vi "Single_ended_2575_DMM_handshake_scan.vi"(0 "resource name":refnum<k15>="R_signal", 1 "resource name":refnum<k15>="DMM", 2 "data path":path, 4 "Scan array":bool[][](array[boolean]), 5 "error in (no error)":errorcluster {"code" format="%.0x"}, 6 "Differential\nMode":bool, 7 "measurement type":T2, 11 "Resolution in Digits":T1=7.5 items=["3 1/2"=3.5, "4 1/2"=4.5, "5 1/2"=5.5, "6 1/2"=6.5, "7 1/2"=7.5], 12 "range":dbl=-1.0 format="%.2f") -> (14 "Measurements 2":dbl[](array[numeric]) caption="Measurements" format="%.7f", 19 "error out":errorcluster {"code" format="%.0x"})   [LabVIEW 2013]
doc: "I. Description:\n\nThis example demonstrates how to scan a series of channels on a switch module and take measurements with an NI digital multimeter using handshaking. \n\nHANDSHAKING:\nFirst, the DMM is initiated and waits for a digital pulse from the switch before taking any measurements. When the switch scanning task is started, it connects the first channel in its scan list, waits for the channel to settle and generates a digital pulse-Scan Advanced. When the DMM receives this digital pulse, it takes the first measurement and generates a digital pulse-Measurement Complete (MC). When the switch receives this digital pulse, it advances to the next entry in its scan list and this continues.\n\nII. Instructions for Running:\n\nTo make this example work with your switch, complete the following:\nSWITCH SETUP: (refer to the NI Switches Help) \nEnter the DAQmx/traditional DAQ switch resource name.\nSelect the correct topology for your switch module.\nEnter a valid scan list.\nSelect valid values for Trigger Input and Scan Advanced Output. \n\nDMM SETUP: (refer to your NI DMM documentation)\nEnter your traditional DAQ DMM resource name.\nSelect measurement type, range and resolution.\nEnter number of samples.\nSelect a valid Measurement Complete Destination and Trigger Source.\n\nRefer to the NI Switches Help to determine if your switch supports scanning, the scan list syntax, and the valid channel names and valid resource names for your switch module.\n\nIII. Block Diagram Steps:\n\nA) The switch is configured first. Triggers and scan list are set. The scanning configuration is downloaded to the hardware with niSwitch Commit.vi.\nB) The DMM is configured. Functions, range, resolution, triggers and number of points to take are set. When the DMM initiates, it configures its hardware according to the settings and waits for a trigger. \nC) When the switch initiates it connects the first channels in its scan list, waits for the relays to settle and send its Scan Advanced signal to trigger the DMM for its first measurement. Once the DMM has taken a measurement, the DMM sends its MC signal to the switch to advance to the next entry in the scan list. \nD) The DMM returns to the user the number of measurements specified in \"Sample to Fetch at a Time\". When the stop button is pushed the acquisition stops.\nE) Terminates the scanning operation, closes the session to the switch, and display errors if any.\n\nIV. I/O Connections Overview:\n\nRefer to the NI Switches Getting Started Guide and NI Switches Help for information about connecting signals to your switch module."
uses:
  <instrlib>/niDMM/nidmm.llb/niDMM Function.ctl
  <instrlib>/niDMM/nidmm.llb/niDMM Trigger.ctl
  <instrlib>/niDMM/nidmm.llb/niDMM Resolution in Digits.ctl
  <instrlib>/niSwitch/niSwitch.LLB/niSwitch Topologies.ctl
  <instrlib>/niDMM/nidmm.llb/niDMM Sample Trigger.ctl
  <instrlib>/niDMM/nidmm.llb/niDMM Configure Measurement Digits.vi
panel:
  in  "trigger source":T3=enum."TTL 2"
  in  "scan advanced output":T4(ring)=enum."TTL2"
  in  "trigger input":T5(ring)=enum."TTL0"
  in  "measurement complete destination":u16(ring)=2 items=["None", "External", "TTL 0", "TTL 1", "TTL 2", "TTL 3", "TTL 4", "TTL 5", "TTL 6", "TTL 7", "LBR Trig 0"]
  out "Measurements":dbl[](graph)=[-0.007577253971248865, -0.007579062599688768, -0.0075269537046551704, -0.007562803104519844]
  # "SWITCH"
  # "DMM"
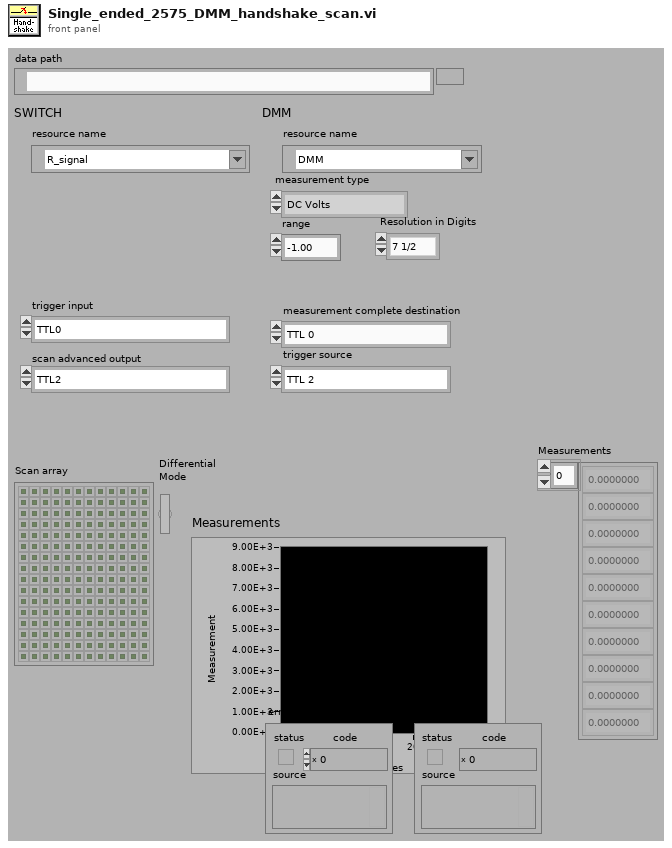
[diagram p1: front panel]
types:
  T1 = typedef "niDMM Resolution in Digits.ctl" = dbl
  T2 = typedef "niDMM Function.ctl" = enum16{"DC Volts", "AC Volts", "DC Current", "AC Current", "2-wire Resistance", "4-wire Resistance", "Diode", "Frequency", "Period", "AC Volts DC Coupled", "Capacitance", "Inductance", "Temperature"}
  T3 = typedef "niDMM Trigger.ctl" = enum16{"Immediate", "External", "TTL 0", "TTL 1", "TTL 2", "TTL 3", "TTL 4", "TTL 5", "TTL 6", "Software", "TTL 7", "PXI Star", "LBR Trig 1", "Aux Trig 1"}
  T4 = enum16{"None", "External", "TTL0", "TTL1", "TTL2", "TTL3", "TTL4", "TTL5", "TTL6", "TTL7", "ECL0", "ECL1", "PXI Star", "Rear Connector", "Front Connector", "Rear Connector Module 1", "Rear Connector Module 2", "Rear Connector Module 3", "Rear Connector Module 4", "Rear Connector Module 5", "Rear Connector Module 6", "Rear Connector Module 7", "Rear Connector Module 8", "Rear Connector Module 9", "Rear Connector Module 10", "Rear Connector Module 11", "Rear Connector Module 12", "Front Connector Module 1", "Front Connector Module 2", "Front Connector Module 3", "Front Connector Module 4", "Front Connector Module 5", "Front Connector Module 6", "Front Connector Module 7", "Front Connector Module 8", "Front Connector Module 9", "Front Connector Module 10", "Front Connector Module 11", "Front Connector Module 12"}
  T5 = enum16{"Immediate", "External", "TTL0", "TTL1", "TTL2", "TTL3", "TTL4", "TTL5", "TTL6", "TTL7", "ECL0", "ECL1", "PXI Star", "Software Trigger Function", "Rear Connector", "Front Connector", "Rear Connector of Module 1", "Rear Connector of Module 2", "Rear Connector of Module 3", "Rear Connector of Module 4", "Rear Connector of Module 5", "Rear Connector of Module 6", "Rear Connector of Module 7", "Rear Connector of Module 8", "Rear Connector of Module 9", "Rear Connector of Module 10", "Rear Connector of Module 11", "Rear Connector of Module 12", "Front Connector of Module 1", "Front Connector of Module 2", "Front Connector of Module 3", "Front Connector of Module 4", "Front Connector of Module 5", "Front Connector of Module 6", "Front Connector of Module 7", "Front Connector of Module 8", "Front Connector of Module 9", "Front Connector of Module 10", "Front Connector of Module 11", "Front Connector of Module 12"}
  T6 = typedef "niSwitch Topologies.ctl" = string
  T7 = typedef "niDMM Sample Trigger.ctl" = enum16{"Immediate", "External", "TTL 0", "TTL 1", "TTL 2", "TTL 3", "TTL 4", "TTL 5", "TTL 6", "Interval", "Software", "TTL 7", "PXI Star", "LBR Trig 1", "Aux Trig 1"}
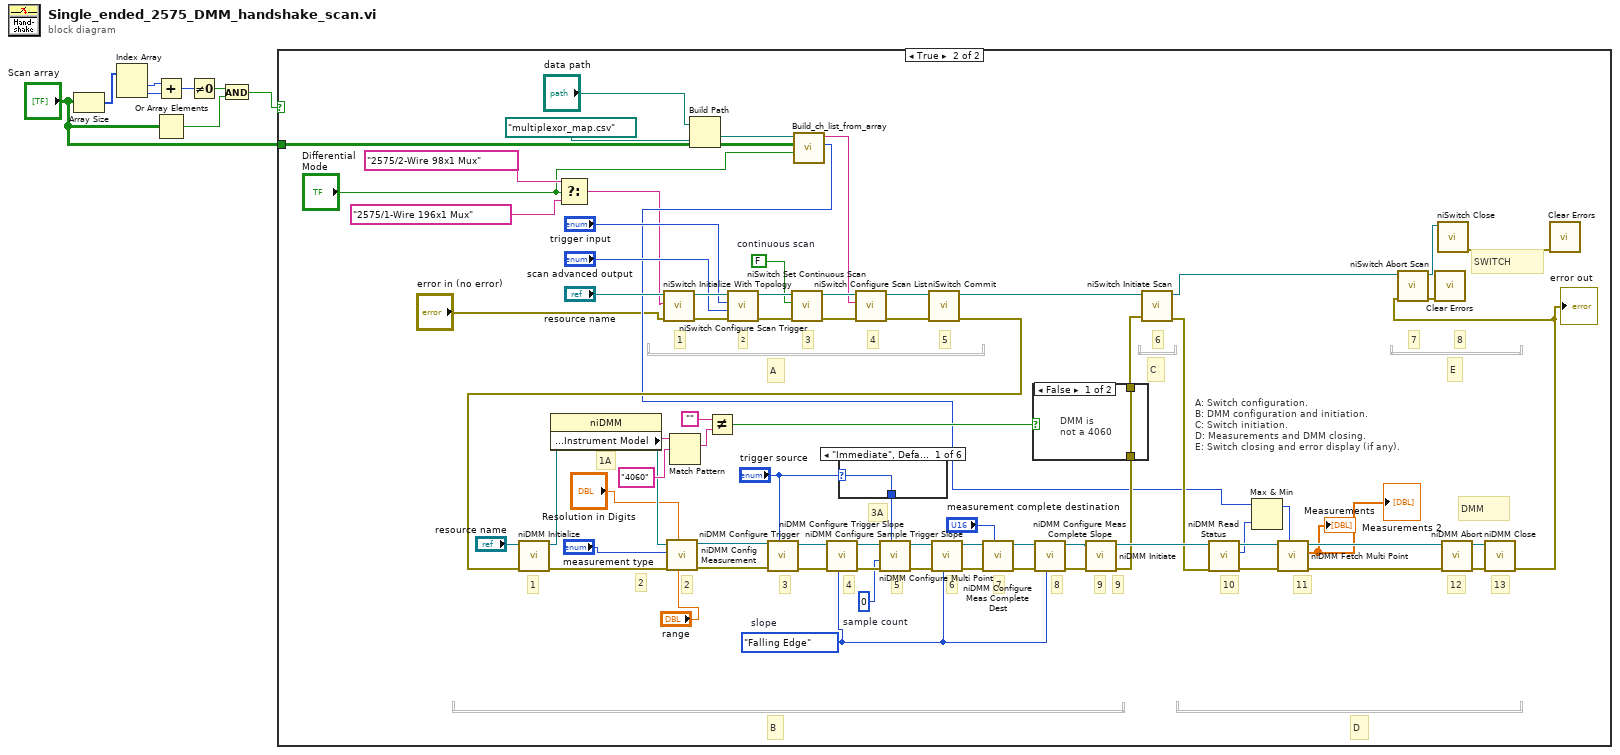
[diagram p0: block diagram]
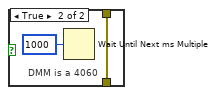
[diagram p3: hidden frame]
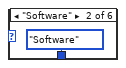
[diagram p4: hidden frame]
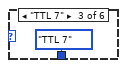
[diagram p5: hidden frame]
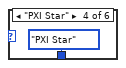
[diagram p6: hidden frame]
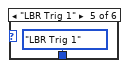
[diagram p7: hidden frame]
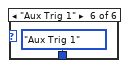
[diagram p8: hidden frame]
diagram:
  n1 = Array Size(array="Scan array") -> (size(s)=w8:i32[])
  n2 = Index Array(array=w8) -> (element #1=w6:i32, element #2=w7:i32)  [unwired: 2 in]
  n3 = Add(x=w6, y=w7) -> (x+y=w5:i32)
  n4 = Or Array Elements(Boolean array="Scan array") -> (logical OR=w1:bool)
  n5 = Not Equal To 0?(x=w5) -> (x != 0?=w4:bool)
  n6 = And(x=w4, y=w1) -> (x .and. y?=w3:bool)
  n7 = case shown="True" w3 {
    tunnel: "Scan array" -> [_ w10]
    frame False {
    }
    frame True {
      w45 = enum16{"Rising Edge", "Falling Edge"}."Falling Edge"  # slope
      w62 = 0  # sample count
      w79 = FALSE  # continuous scan
      # "11"
      # "10"
      # "9"
      # "2"
      # "5"
      # "9"
      # "13"
      # "12"
      # "8"
      # "B"
      # "3A"
      # "1A"
      # "4"
      # "6"
      # "5"
      # "7"
      # "3"
      # "2"
      # "1"
      # "E"
      # "D"
      # "C"
      # "A"
      # "DMM"
      # "SWITCH"
      # "6"
      # "8"
      # "7"
      # "4"
      # "3"
      # "2"
      # "1"
      # "A: Switch configuration.\nB: DMM configuration and initiation.\nC: Switch initiation.\nD: Measurements and DMM closing.\nE: Switch closing and error display (if any)."
      n8 = Select(t=T6 "2575/2-Wire 98x1 Mux" ("topology name"), s="Differential\nMode", f=T6 "2575/1-Wire 196x1 Mux" ("topology name")) -> (s? t:f=w13:T6)
      n9 = call <instrlib>:"niSwitch Initialize With Topology.vi"("error in (no error)"="error in (no error)", "topology name"=w13, "resource name"="resource name") -> ("error out"=w76:errorcluster, "instrument handle out"=w77:refnum<k15>)  [unwired: 7 in]
      n10 = Build Path(base path="data path", name or relative path=path "multiplexor_map.csv" ("Ch definition path (dialog if empty)")) -> (appended path=w11:path)
      n11 = call <instrlib>:"niSwitch Configure Scan Trigger.vi"("error in (no error)"=w76, "scan advanced output (External)"="scan advanced output", "trigger input (External)"="trigger input", "instrument handle"=w77) -> ("error out"=w80:errorcluster, "instrument handle out"=w82:refnum<k15>)  [unwired: 6 in]
      n12 = call <instrlib>:"niSwitch Set Continuous Scan.vi"("error in (no error)"=w80, "continuous scan (False)"=w79, "instrument handle"=w82) -> ("error out"=w74:errorcluster, "instrument handle out"=w75:refnum<k15>)  [unwired: 7 in]
      n13 = call "Build_ch_list_from_array.vi"("Differential\nMode"="Differential\nMode", "Scan array"=w10, "Ch definition path (dialog if empty)"=w11) -> ("number of contacts"=w27:i32, "Scan String"=w28:string)  [unwired: 7 in]
      n14 = case shown="\"Immediate\", Default" "trigger source" {
        selector: "trigger source" -> [w86 _ _ _ _ _]
        tunnel: [w86 niDMM_Sample_Trigger."Software" ("Sample Trigger") niDMM_Sample_Trigger."TTL 7" ("Sample Trigger") niDMM_Sample_Trigger."PXI Star" ("Sample Trigger") niDMM_Sample_Trigger."LBR Trig 1" ("Sample Trigger") niDMM_Sample_Trigger."Aux Trig 1" ("Sample Trigger")] -> w59
        frame "Immediate", Default {
        }
        frame "Software" {
        }
        frame "TTL 7" {
        }
        frame "PXI Star" {
        }
        frame "LBR Trig 1" {
        }
        frame "Aux Trig 1" {
        }
      }
      n15 = call <instrlib>:"niSwitch Configure Scan List.vi"("error in (no error)"=w74, "scan list"=w28, "instrument handle"=w75) -> ("error out"=w39:errorcluster, "instrument handle out"=w38:refnum<k15>)  [unwired: 7 in]
      n16 = call <instrlib>:"niSwitch Commit.vi"("error in (no error)"=w39, "instrument handle"=w38) -> ("error out"=w37:errorcluster, "instrument handle out"=w20:refnum<k15>)  [unwired: 8 in]
      n17 = call <instrlib>:"niDMM Initialize.vi"("error in (no error)"=w37, "Instrument Descriptor"="resource name") -> ("error out"=w33:errorcluster, "instrument handle out"=w40:refnum<k15>)  [unwired: 8 in]
      n18 = property class="niDMM"(reference=w40) -> (reference out=w35:refnum<k15>, "Inherent IVI Attributes:Instrument Identification:Instrument Model"=w41:string)  [unwired: 1 in, 1 out]
      n19 = call-poly <instrlib>:"niDMM Config Measurement.vi"("Range"="range", "Resolution in Digits"="Resolution in Digits", "error in (no error)"=w33, "Function"="measurement type", "instrument handle"=w35) -> ("error out"=w30:errorcluster, "instrument handle out"=w31:refnum<k15>)  [unwired: 5 in]
      n20 = Match Pattern(string=w41, regular expression="4060") -> (match substring=w56:string)  [unwired: 1 in, 3 out]
      n21 = Not Equal?(x="", y=w56) -> (x != y?=w54:bool)
      n22 = call <instrlib>:"niDMM Configure Trigger.vi"("Trigger Source"="trigger source", "error in (no error)"=w30, "instrument handle"=w31) -> ("error out"=w67:errorcluster, "instrument handle out"=w68:refnum<k15>)  [unwired: 7 in]
      n23 = call <instrlib>:"niDMM Configure Trigger Slope.vi"("Slope"=w45, "error in (no error)"=w67, "instrument handle"=w68) -> ("error out"=w65:errorcluster, "instrument handle out"=w66:refnum<k15>)  [unwired: 7 in]
      n24 = call <instrlib>:"niDMM Configure Multi Point.vi"("Sample Trigger"=w59, "error in (no error)"=w65, "Sample Count"=w62, "instrument handle"=w66) -> ("error out"=w63:errorcluster, "instrument handle out"=w64:refnum<k15>)  [unwired: 6 in]
      n25 = call <instrlib>:"niDMM Configure Sample Trigger Slope.vi"("Slope"=w45, "error in (no error)"=w63, "instrument handle"=w64) -> ("error out"=w52:errorcluster, "instrument handle out"=w51:refnum<k15>)  [unwired: 7 in]
      n26 = call <instrlib>:"niDMM Configure Meas Complete Dest.vi"("Measurement Complete Destination"="measurement complete destination", "error in (no error)"=w52, "instrument handle"=w51) -> ("error out"=w46:errorcluster, "instrument handle out"=w49:refnum<k15>)  [unwired: 7 in]
      n27 = call <instrlib>:"niDMM Configure Meas Complete Slope.vi"("Slope"=w45, "error in (no error)"=w46, "instrument handle"=w49) -> ("error out"=w47:errorcluster, "instrument handle out"=w48:refnum<k15>)  [unwired: 7 in]
      n28 = call <instrlib>:"niDMM Initiate.vi"("error in (no error)"=w47, "instrument handle"=w48) -> ("error out"=w58:errorcluster, "instrument handle out"=w72:refnum<k15>)  [unwired: 8 in]
      n29 = case shown="False" w54 {
        tunnel: w58 -> [w83 w84]
        tunnel: [w83 w84] -> w53
        frame False {
          # "DMM is \nnot a 4060"
        }
        frame True {
          # "DMM is a 4060"
          n30 = Wait Until Next ms Multiple(millisecond multiple=u32 1000) -> ()  [unwired: 1 out]
        }
      }
      n31 = call <instrlib>:"niSwitch Initiate Scan.vi"("error in (no error)"=w53, "instrument handle"=w20) -> ("error out"=w44:errorcluster, "instrument handle out"=w73:refnum<k15>)  [unwired: 8 in]
      n32 = call <instrlib>:"niDMM Read Status.vi"("error in (no error)"=w44, "instrument handle"=w72) -> ("error out"=w26:errorcluster, "Backlog"=w24:i32, "instrument handle out"=w25:refnum<k15>)  [unwired: 6 in, 1 out]
      n33 = Max & Min(x=w27, y=w24) -> (max(x,y)=w23:i32)  [unwired: 1 out]
      n34 = call <instrlib>:"niDMM Fetch Multi Point.vi"("Number to Fetch"=w23, "error in (no error)"=w26, "instrument handle"=w25) -> ("error out"=w61:errorcluster, "Measurements"=→"Measurements" →"Measurements 2":dbl[], "instrument handle out"=w60:refnum<k15>)  [unwired: 5 in, 1 out]
      n35 = call <instrlib>:"niDMM Abort.vi"("error in (no error)"=w61, "instrument handle"=w60) -> ("error out"=w70:errorcluster, "instrument handle out"=w71:refnum<k15>)  [unwired: 8 in]
      n36 = call <instrlib>:"niDMM Close.vi"("error in (no error)"=w70, "instrument handle"=w71) -> ("error out"=w17:errorcluster)  [unwired: 9 in]
      "error out" <- w17
      n37 = call <instrlib>:"niSwitch Abort Scan.vi"("error in (no error)"=w17, "instrument handle"=w73) -> ("error out"=w19:errorcluster, "instrument handle out"=w81:refnum<k15>)  [unwired: 8 in]
      n38 = call <vilib>:"Clear Errors.vi"("error in (no error)"=w19) -> ()  [unwired: 6 in, 1 out]
      n39 = call <instrlib>:"niSwitch Close.vi"("instrument handle"=w81) -> ("error out"=w18:errorcluster)  [unwired: 10 in]
      n40 = call <vilib>:"Clear Errors.vi"("error in (no error)"=w18) -> ()  [unwired: 6 in, 1 out]
    }
  }
